vi "Start Aquisition.vi"(8 "error in (no error)":errorcluster, 10 "Camera":string, 11 "HIJ Vision Camera App in":refnum<class "HIJ Vision Camera App.lvclass">) -> (0 "error out":errorcluster, 3 "HIJ Vision Camera App out":refnum<class "HIJ Vision Camera App.lvclass">)   [LabVIEW 2014, in "HIJ Vision Camera App.lvlib" / "HIJ Vision Camera App.lvclass"]
uses:
  HIJ Vision Camera App.lvclass
  HIJ Vision Camera App.lvclass/HIJ Vision Camera App.ctl
  Camera Actor/Camera Actor Messages/Start Acquisition Msg/Start Acquisition Msg.lvclass/Start Acquisition Msg.ctl
  <vilib>/ActorFramework/Message Enqueuer/Message Enqueuer.lvclass/Message Enqueuer.ctl
  HIJ Vision Application/HIJ Vision Application/HIJ Vision Application.lvclass/HIJ Vision Application.ctl
  HIJ Vision Display/HIJ Vision Display Messages/Change Image Source Msg/Change Image Source Msg.lvclass/Change Image Source Msg.ctl
  HIJ Vision Application/HIJ Vision Application/Read Display Enq.vi
  <vilib>/ActorFramework/Message Enqueuer/Enqueue.vi
  <vilib>/ActorFramework/Message Priority Queue/Priority Enqueue.vi
  Camera Actor/Camera Actor Messages/Start Acquisition Msg/Start Acquisition Msg.lvclass
  <vilib>/ActorFramework/Message Enqueuer/Message Enqueuer.lvclass
  HIJ Vision Display/HIJ Vision Display Messages/Change Image Source Msg/Change Image Source Msg.lvclass
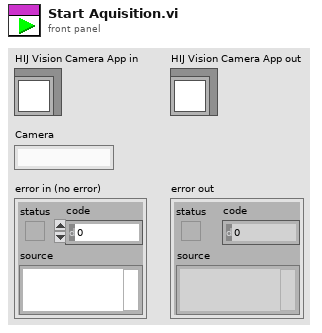
[diagram p1: front panel]
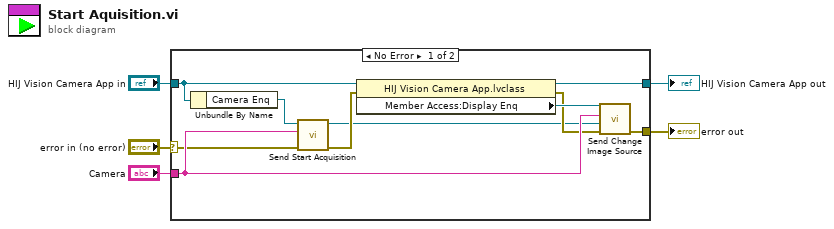
[diagram p0: block diagram]
diagram:
  n1 = case shown="No Error" "error in (no error)" {
    selector: "error in (no error)" -> [w13 w17]
    tunnel: [w11 w17] -> w4
    tunnel: [w8 w16] -> w2
    tunnel: "HIJ Vision Camera App in" -> [w9 w16]
    tunnel: "Camera" -> [w15 _]
    frame No Error {
      n2 = Unbundle By Name(w9) -> ("Camera Enq"=w14:refnum<class "Message Enqueuer.lvclass">)
      n3 = call "Send Start Acquisition.vi"("error in (no error)"=w13, "Camera Name"=w15, "Message Enqueuer"=w14) -> ("error out"=w12:errorcluster, "Message Enqueuer out"=w6:refnum<class "Message Enqueuer.lvclass">)  [unwired: 7 in]
      n4 = property class="HIJ Vision Camera App.lvclass"(reference=w9, error in=w12) -> (reference out=w8:refnum<class "HIJ Vision Camera App.lvclass">, error out=w7:errorcluster, "Member Access:Display Enq"=w10:refnum<class "Message Enqueuer.lvclass">)
      n5 = call "Send Change Image Source.vi"("error in (no error)"=w7, "Image Source Enq"=w6, "Image Source"=w15, "Message Enqueuer"=w10) -> ("error out"=w11:errorcluster)  [unwired: 6 in, 1 out]
    }
    frame Error {
    }
  }
  "error out" <- w4
  "HIJ Vision Camera App out" <- w2
